vi "SR400 GetGateParams.vi"(8 "error in (no error)":errorcluster, 11 "VISA Port In":refnum<visa-resource-name>="GPIB0::23::INSTR") -> (0 "error out":errorcluster, 1 "BGatePar":T1={"Mode"=0, "Durée"=0.9992, "Délais"=0.9992, "Incrément"=0.9992} caption="Paramètres de la porte d'acquisition «B»" {"Incrément" min=0.0 max=0.9992 step=1e-09 format="%#_4g"; "Délais" min=0.0 max=0.9992 step=1e-09 format="%#_4g"; "Durée" min=5e-09 max=0.9992 step=1e-09 format="%#_4g"; "Mode" items=["CW", "Fixed", "Scan"]}, 2 "AGatePar":T1={"Mode"=0, "Durée"=0.9992, "Délais"=0.9992, "Incrément"=0.9992} caption="Paramètres de la porte d'acquisition «A»" {"Incrément" min=0.0 max=0.9992 step=1e-09 format="%#_4g"; "Délais" min=0.0 max=0.9992 step=1e-09 format="%#_4g"; "Durée" min=5e-09 max=0.9992 step=1e-09 format="%#_4g"; "Mode" items=["CW", "Fixed", "Scan"]}, 3 "VISA Port Out":refnum<visa-resource-name>="SR400")   [LabVIEW 2012]
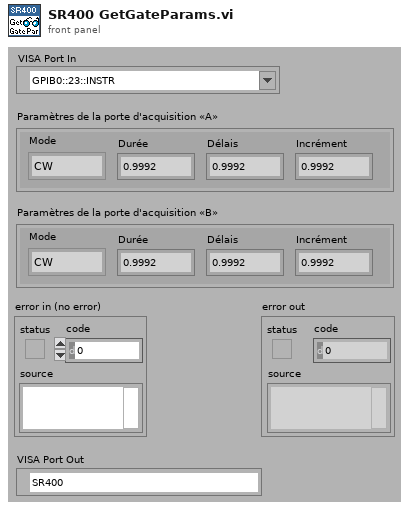
[diagram p1: front panel]
types:
  T1 = cluster{"Mode":u16, "Durée":dbl, "Délais":dbl, "Incrément":dbl}
  T2 = enum16{"Lit le Statut", "Demande Param", "Lit Param", "Oper. incomp."}
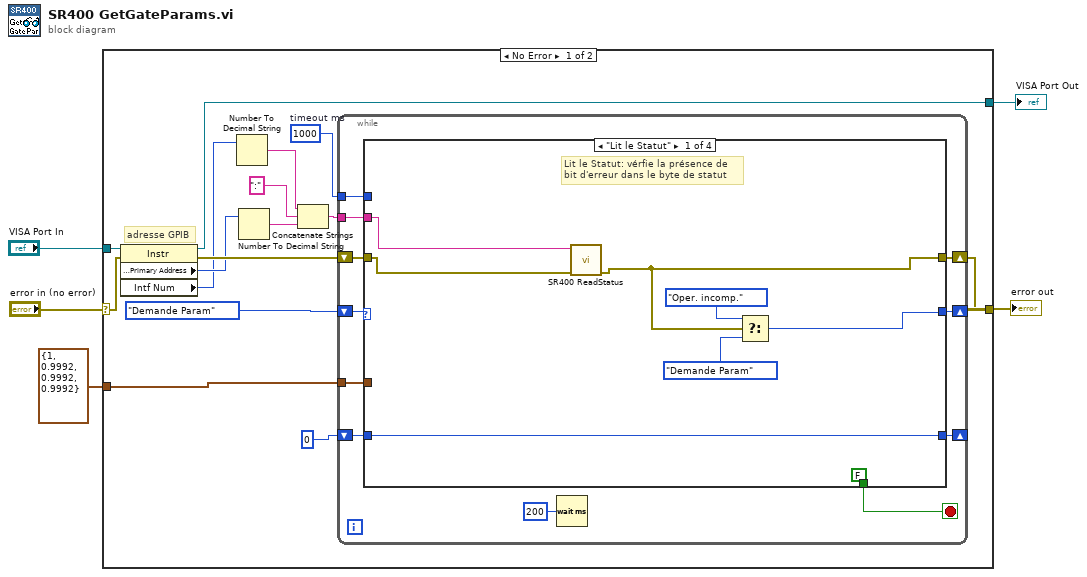
[diagram p0: block diagram]
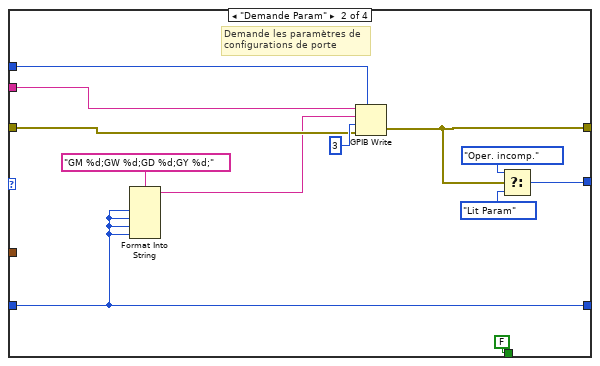
[diagram p2: hidden frame]
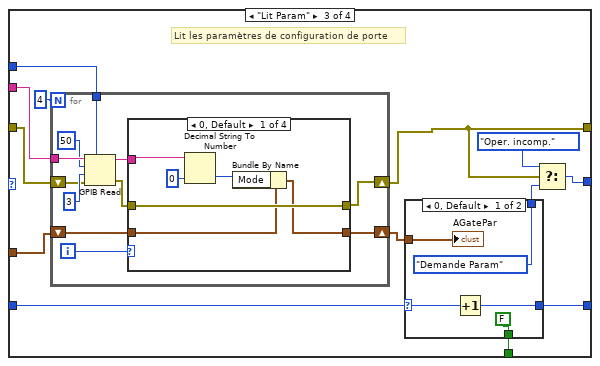
[diagram p3: hidden frame]
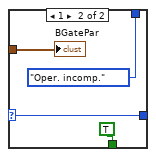
[diagram p4: hidden frame]
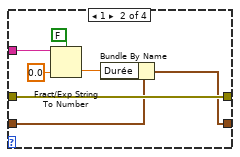
[diagram p5: hidden frame]
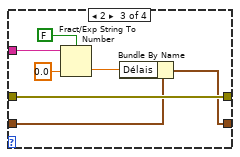
[diagram p6: hidden frame]
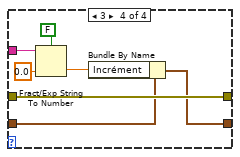
[diagram p7: hidden frame]
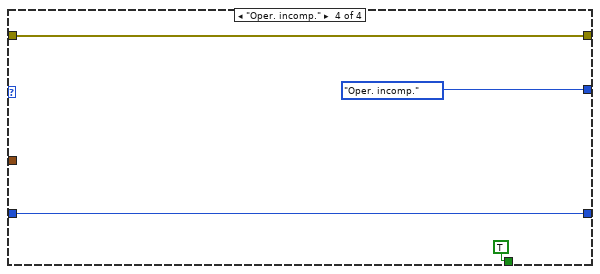
[diagram p8: hidden frame]
diagram:
  n1 = case shown="No Error" "error in (no error)" {
    selector: "error in (no error)" -> [w20 w117]
    tunnel: [w14 w117] -> w4
    tunnel: "VISA Port In" -> [w19 w116]
    tunnel: T1 {"Mode"=1, "Durée"=0.9992, "Délais"=0.9992, "Incrément"=0.9992} ("AGatePar") -> [w13 _]
    tunnel: [w6 w116] -> w1
    frame No Error {
      w15 = 1000  # timeout ms
      # "adresse GPIB"
      n2 = property class="Instr"(reference=w19, error in=w20) -> (reference out=w6:refnum<visa-resource-name>, error out=w18:errorcluster, "GPIB Settings:Primary Address"=w16:u16, "Intf Num"=w11:u16)
      n3 = Number To Decimal String(number=w11) -> (decimal integer string=w9:string)  [unwired: 1 in]
      n4 = Number To Decimal String(number=w16) -> (decimal integer string=w8:string)  [unwired: 1 in]
      n5 = Concatenate Strings(w9, ":" ("string"), w8) -> (w10:string)
      n6 = while {
        shift-right: [w25] -> _
        shift-left: T2."Demande Param" -> [w31]
        tunnel: w10 -> [w29]
        shift-right: [w28] -> w14
        shift-left: w18 -> [w30]
        tunnel: w15 -> [w27]
        tunnel: w13 -> [w23]
        shift-right: [w21] -> _
        shift-left: 0 -> [w22]
        stop <- w26 stop-if-true
        n7 = case shown="\"Lit le Statut\"" w31 {
          tunnel: w30 -> [w38 w50 w63 w115]
          tunnel: w29 -> [w37 w49 w64 _]
          tunnel: [w32 w40 w52 w115] -> w28
          tunnel: w27 -> [_ w48 w53 _]
          tunnel: [FALSE ("Configuration\neffectuée") FALSE ("Configuration\neffectuée") w59 TRUE ("Configuration\neffectuée")] -> w26
          tunnel: [w36 w46 w56 T2."Oper. incomp."] -> w25
          tunnel: w23 -> [_ _ w61 _]
          tunnel: w22 -> [w33 w42 w60 w112]
          tunnel: [w33 w42 w55 w112] -> w21
          frame "Lit le Statut" {
            # "Lit le Statut: vérfie la présence de bit d'erreur dans le byte de statut"
            n8 = call <userlib>:"SR400 ReadStatus.vi"("error in"=w38, "Address string"=w37) -> ("Error Out"=w32:errorcluster)  [unwired: 6 in, 1 out]
            n9 = Select(t=T2."Oper. incomp.", s=w32, f=T2."Demande Param") -> (s? t:f=w36:T2)
          }
          frame "Demande Param" {
            # "Demande les paramètres de configurations de porte"
            n10 = Format Into String(format string="GM %d;GW %d;GD %d;GY %d;", w42, w42, w42, w42) -> (resulting string=w41:string)  [unwired: 2 in, 1 out]
            n11 = GPIB Write(0:w49, 1:w41, 2:i16 3 ("mode (0)"), 3:w50, 4:w48) -> (6:w40:errorcluster)  [unwired: 1 out]
            n12 = Select(t=T2."Oper. incomp.", s=w40, f=T2."Lit Param") -> (s? t:f=w46:T2)
          }
          frame "Lit Param" {
            # "Lit les paramètres de configuration de porte"
            n13 = for {
              N: 4 -> [_]
              tunnel: w64 -> [w84]
              shift-right: [w77] -> w52
              shift-left: w63 -> [w81]
              shift-right: [w75] -> w54
              shift-left: w61 -> [w76]
              tunnel: w53 -> [w74]
              i -> [w80]
              n14 = GPIB Read(0:w84, 1:50 ("byte count"), 2:i16 3 ("mode (0)"), 3:w81, 4:w74) -> (5:w79:string, 7:w78:errorcluster)  [unwired: 1 out]
              n15 = case shown="0, Default" w80 {
                tunnel: w79 -> [w90 w96 w103 w110]
                tunnel: w78 -> [w88 w95 w102 w109]
                tunnel: [w88 w95 w102 w109] -> w77
                tunnel: w76 -> [w87 w92 w99 w106]
                tunnel: [w86 w91 w98 w105] -> w75
                frame 0, Default {
                  n16 = Decimal String To Number(string=w90, default (0L)=u16 0 ("default (0 I32)")) -> (number=w85:u16)  [unwired: 1 in, 1 out]
                  n17 = Bundle By Name(cluster=w87, "Mode"=w85) -> (w86:T1)
                }
                frame 1 {
                  n18 = Fract/Exp String To Number(use system decimal point (T)=FALSE, string=w96, default (0 dbl)=0.0 ("default (0 I32)")) -> (number=w93:dbl)  [unwired: 1 in, 1 out]
                  n19 = Bundle By Name(cluster=w92, "Durée"=w93) -> (w91:T1)
                }
                frame 2 {
                  n20 = Fract/Exp String To Number(use system decimal point (T)=FALSE, string=w103, default (0 dbl)=0.0 ("default (0 I32)")) -> (number=w100:dbl)  [unwired: 1 in, 1 out]
                  n21 = Bundle By Name(cluster=w99, "Délais"=w100) -> (w98:T1)
                }
                frame 3 {
                  n22 = Fract/Exp String To Number(use system decimal point (T)=FALSE, string=w110, default (0 dbl)=0.0 ("default (0 I32)")) -> (number=w107:dbl)  [unwired: 1 in, 1 out]
                  n23 = Bundle By Name(cluster=w106, "Incrément"=w107) -> (w105:T1)
                }
              }
            }
            n24 = case shown="0, Default" w60 {
              selector: w60 -> [w67 w71]
              tunnel: [FALSE ("Configuration\neffectuée") TRUE ("Configuration\neffectuée")] -> w59
              tunnel: [T2."Demande Param" T2."Oper. incomp."] -> w57
              tunnel: [w66 w71] -> w55
              tunnel: w54 -> [w65 w70]
              frame 0, Default {
                n25 = Increment(x=w67) -> (x+1=w66:i32)
                "AGatePar" <- w65
              }
              frame 1 {
                "BGatePar" <- w70
              }
            }
            n26 = Select(t=T2."Oper. incomp.", s=w52, f=w57) -> (s? t:f=w56:T2)
          }
          frame "Oper. incomp." {
          }
        }
        n27 = Wait (ms)(milliseconds to wait=u32 200) -> ()  [unwired: 1 out]
      }
    }
    frame Error {
    }
  }
  "error out" <- w4
  "VISA Port Out" <- w1
